vi "Chip with NanoStructures.vi"(4 "Length of Chip":dbl, 5 "NS Base Area":dbl, 6 "m-nm WChip":dbl, 7 "NS Length":dbl, 8 "Width of Chip":dbl, 9 "Gap n-m":dbl, 10 "m-nm LChip":dbl, 11 "Gap B/W NS":dbl) -> (0 "Gap B/w NS":dbl, 3 "No of NS Pairs on Chip":dbl)   [LabVIEW 2020]
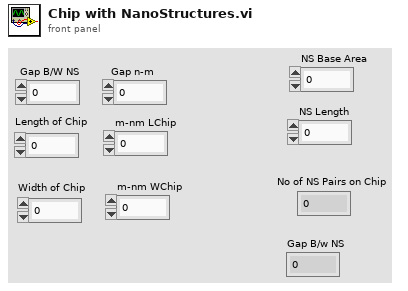
[diagram p1: front panel]
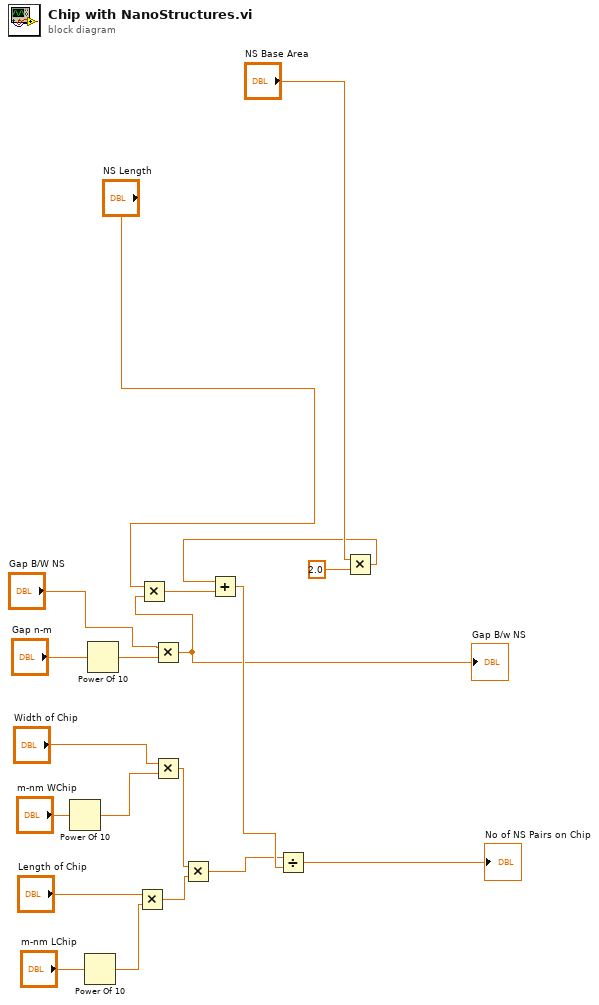
[diagram p0: block diagram]
diagram:
  n1 = Power Of 10(x="m-nm WChip") -> (10^x=w2:dbl)
  n2 = Power Of 10(x="m-nm LChip") -> (10^x=w6:dbl)
  n3 = Power Of 10(x="Gap n-m") -> (10^x=w11:dbl)
  n4 = Multiply(x="Length of Chip", y=w6) -> (x*y=w7:dbl)
  n5 = Multiply(x="Gap B/W NS", y=w11) -> (x*y=w13:dbl)
  "Gap B/w NS" <- w13
  n6 = Multiply(x="NS Length", y=w13) -> (x*y=w14:dbl)
  n7 = Multiply(x="Width of Chip", y=w2) -> (x*y=w8:dbl)
  n8 = Multiply(x=w8, y=w7) -> (x*y=w9:dbl)
  n9 = Multiply(x="NS Base Area", y=2.0) -> (x*y=w18:dbl)
  n10 = Add(x=w18, y=w14) -> (x+y=w15:dbl)
  n11 = Divide(x=w9, y=w15) -> (x/y=→"No of NS Pairs on Chip":dbl)
